vi "Update Board Info.vi"(0 "Input Parsed":T1, 5 "Array":string[](array[string]), 11 "error in (no error)":errorcluster) -> (4 "Input Parsed":T1, 15 "error out":errorcluster)   [LabVIEW 2014, in "Dragon Tamers.lvlib"]
uses:
  Dragon Tamers.lvlib
  Typedefs/Input Parsed.ctl
  Typedefs/King.ctl
  Typedefs/Cell Pos.ctl
  Typedefs/Board.ctl
  Typedefs/Board Cell.ctl
  Typedefs/Cell Occupancy.ctl
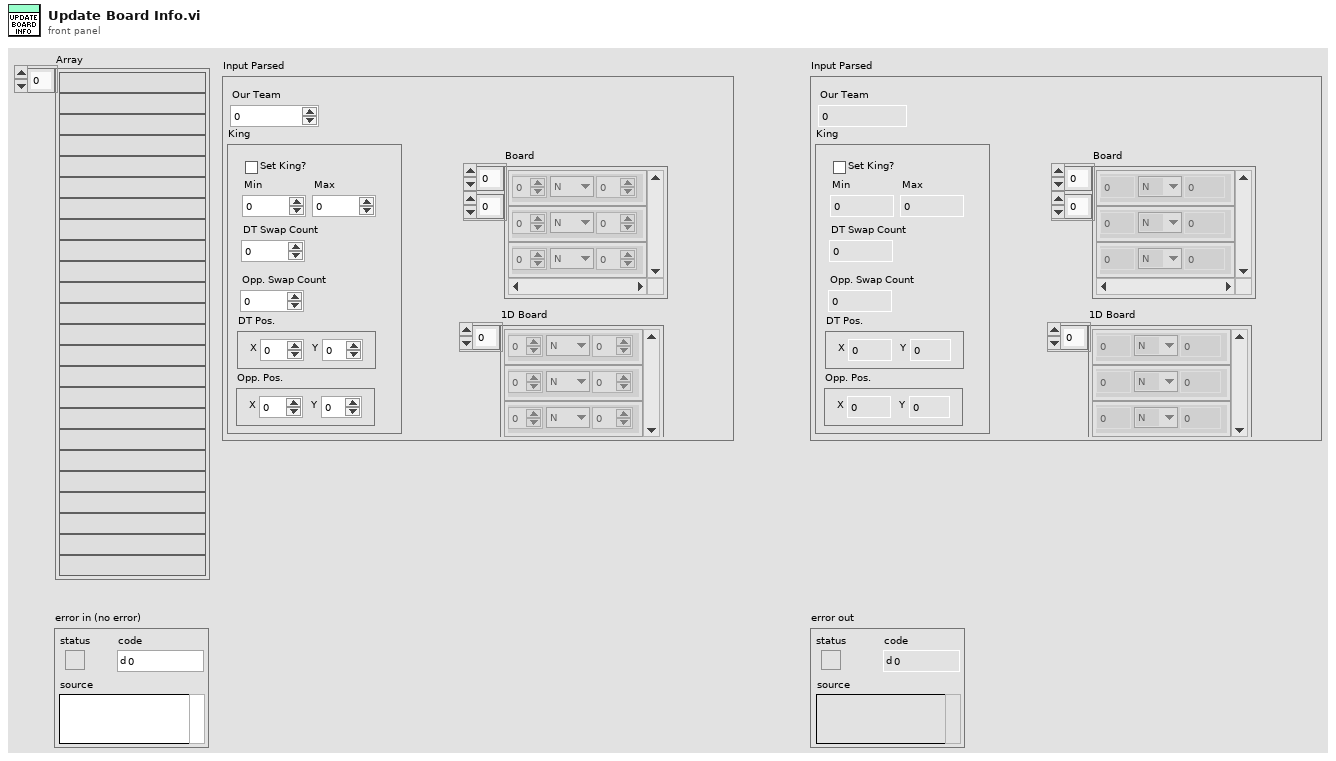
[diagram p1: front panel]
types:
  T1 = typedef "Dragon Tamers.lvlib/Input Parsed.ctl" = cluster{"Our Team":i32, "King":T2, "Board":T4, "1D Board":T5[]}
  T2 = typedef "Dragon Tamers.lvlib/King.ctl" = cluster{"Set King?":bool, "Min":i32, "Max":i32, "DT Swap Count":i32, "Opp. Swap Count":i32, "DT Pos.":T3, "Opp. Pos.":T3}
  T3 = typedef "Dragon Tamers.lvlib/Cell Pos.ctl" = cluster{"X":i32, "Y":i32}
  T4 = typedef "Dragon Tamers.lvlib/Board.ctl" = T5[][]
  T5 = typedef "Dragon Tamers.lvlib/Board Cell.ctl" = cluster{"Team":i32, "Occu.":T6, "Count":i32}
  T6 = typedef "Dragon Tamers.lvlib/Cell Occupancy.ctl" = enum16{"N", "C", "K"}
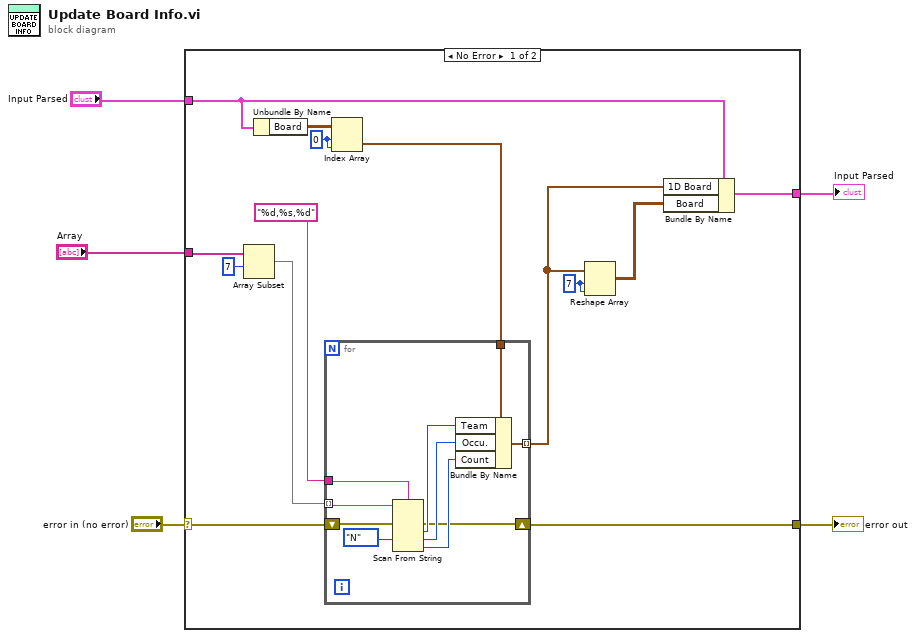
[diagram p0: block diagram]
diagram:
  n1 = case shown="No Error" "error in (no error)" {
    selector: "error in (no error)" -> [w7 w30]
    tunnel: [w6 w30] -> w4
    tunnel: "Array" -> [w19 _]
    tunnel: "Input Parsed" -> [w14 _]
    tunnel: [w9 _] -> w1
    frame No Error {
      w13 = 0 ("index (row)")
      w15 = 7 ("dimension size")
      n2 = Array Subset(array=w19, index=7) -> (w17:string[])  [unwired: 1 in]
      n3 = Unbundle By Name(w14) -> ("Board"=w12:T4)
      n4 = Index Array(array=w12, index (row)=w13, index (col)=w13) -> (element=w11:T5)
      n5 = for {
        tunnel: w17 -> [w29] mode=indexing
        tunnel: "%d,%s,%d" ("format string") -> [w28]
        tunnel: [w23] -> w8 mode=indexing
        tunnel: w11 -> [w22]
        shift-right: [w20] -> w6
        shift-left: w7 -> [w21]
        n6 = Scan From String(format string=w28, input string=w29, error in=w21, default 2=Cell_Occupancy."N" ("Occupancy")) -> (error out=w20:errorcluster, output 1=w26:i32, output 2=w25:T6, output 3=w24:i32)  [unwired: 3 in, 2 out]
        n7 = Bundle By Name(cluster=w22, "Team"=w26, "Occu."=w25, "Count"=w24) -> (w23:T5)
      }
      n8 = Reshape Array(w8, w15, w15) -> (w10:T5[][])
      n9 = Bundle By Name(cluster=w14, "1D Board"=w8, "Board"=w10) -> (w9:T1)
    }
    frame Error {
    }
  }
  "error out" <- w4
  "Input Parsed" <- w1
